vi "Global TS.vi"() -> ()   [LabVIEW 2023, in "GUI.lvlib"]
uses:
  GUI.lvlib
panel:
  in  "Globals":refnum<k7>
  in  "Thread":refnum<k7>
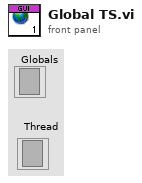
[diagram p1: front panel]
diagram:
